vi "Find Custom Device by Name.vi"(8 "error in (no error)":errorcluster, 10 "Name":string, 11 "Target in":refnum<k24>) -> (0 "error out":errorcluster, 2 "CD Ref":T1 format="%.0x", 3 "Target out":refnum<k24>)   [LabVIEW 2017, in "Switch Scripting.lvlib"]
uses:
  Switch Scripting.lvlib
  NationalInstruments.VeriStand.SystemDefinitionAPI
  <vilib>/NI Veristand/Custom Device API/Custom Device Item Ref.ctl
  <vilib>/NI VeriStand/Custom Device API/Custom Device API.lvlib
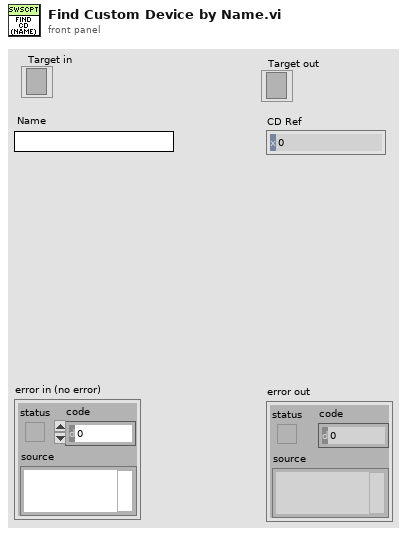
[diagram p1: front panel]
types:
  T1 = typedef "Custom Device API.lvlib/Custom Device Item Ref.ctl" = u64
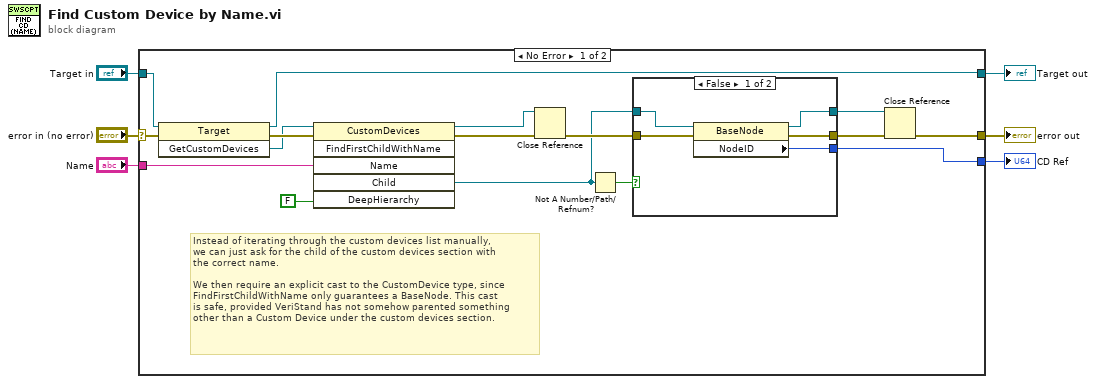
[diagram p0: block diagram]
diagram:
  n1 = case shown="No Error" "error in (no error)" {
    selector: "error in (no error)" -> [w22 w31]
    tunnel: [w8 w31] -> w6
    tunnel: "Target in" -> [w21 w30]
    tunnel: [w13 w30] -> w3
    tunnel: "Name" -> [w17 _]
    tunnel: [w10 _] -> w1
    frame No Error {
      # "Instead of iterating through the custom devices list manually,\nwe can just ask for the child of the custom devices section with\nthe correct name.\n\nWe then require an explicit cast to the CustomDevice type, since\nFindFirstChildWithName only guarantees a BaseNode. This cast\nis safe, provided VeriStand has not somehow parented something\nother than a Custom Device under the custom devices section."
      n2 = invoke class="Target" method="GetCustomDevices"(reference=w21, error in=w22) -> (reference out=w13:refnum<k24>, error out=w20:errorcluster, "GetCustomDevices"=w19:refnum<k24>)  [unwired: 1 in]
      n3 = invoke class="CustomDevices" method="FindFirstChildWithName"(reference=w19, error in=w20, "Name"=w17, "DeepHierarchy"=FALSE) -> (reference out=w16:refnum<k24>, error out=w15:errorcluster, "Child"=w12:refnum<k24>)  [unwired: 2 in, 3 out]
      n4 = Close Reference(reference=w16, error in (no error)=w15) -> (error out=w14:errorcluster)
      n5 = Not A Number/Path/Refnum?(number/path/refnum=w12) -> (NaN/Path/Refnum?=w11:bool)
      n6 = case shown="False" w11 {
        tunnel: [w23 w29] -> w7
        tunnel: w14 -> [w25 w29]
        tunnel: w12 -> [w27 w28]
        tunnel: [w26 _] -> w10
        tunnel: [w24 w28] -> w9
        frame False {
          n7 = property class="BaseNode"(reference=w27, error in=w25) -> (reference out=w24:refnum<k24>, error out=w23:errorcluster, "NodeID"=w26:u64)
        }
        frame True {
        }
      }
      n8 = Close Reference(reference=w9, error in (no error)=w7) -> (error out=w8:errorcluster)
    }
    frame Error {
    }
  }
  "Target out" <- w3
  "error out" <- w6
  "CD Ref" <- w1
